vi "Process.vi"(8 "error in":errorcluster, 11 "Inst.Transport in":refnum<class "Inst.Transport.lvclass">) -> (0 "error out":errorcluster, 3 "Inst.Transport out":refnum<class "Inst.Transport.lvclass">)   [LabVIEW 2019, in "Inst.Transport.lvclass"]
doc: "---------------------------------------------------------------\nJKI State Machine Objects™\nhttp://jki.net/state-machine-objects/\nCopyright (C) 2005-2015, JKI <info@jki.net>\nALL RIGHTS RESERVED"
uses:
  Inst.Transport.lvclass
  C:/Program Files/National Instruments/LabVIEW 2019/vi.lib/JKI/JKI SMO/SMO/SMO.lvclass
  C:/Program Files/National Instruments/LabVIEW 2019/user.lib/LevyLab/Instrument Framework/Instrument/Instrument.lvclass
  Transport/Typedefs/Lockin_Sweep JSON--Cluster.ctl
  Transport/Transport.lvclass/Transport.ctl
  Typedefs/UI State--enum.ctl
  Typedefs/Inst.Transport.PublicCommands--Enum.ctl
  Typedefs/Inst.Transport.ProtectedCommands--Enum.ctl
  Typedefs/startTransport--Request--Cluster.ctl
  Transport/Typedefs/Transport.Methods--Enum.ctl
  Typedefs/PrivateEvents--MessageToProcess.ctl
  <userlib>/LevyLab/RemoteControl/RemoteControl/Typedefs/Message--Cluster.ctl
  Typedefs/Inst.Transport.Status--Enum.ctl
  Inst.Transport.lvclass/Inst.Transport.ctl
  <vilib>/JKI/JKI SMO/SMO/SMO.lvclass/SMO.ctl
  Control Experiment/Control Experiment.lvclass
  Control Experiment/Control Experiment.lvclass/Control Experiment.ctl
  Typedefs/RefreshTime--Request--Cluster.ctl
  8f0a8fc2-545a-492d-a380-fe326c3f5926.vi
  1045582e-a15c-4059-9878-8d398bb7fea9.vi
  db7760a1-0849-494e-b918-bfd2b1278472.vi
  48eb5b5f-56a5-4c0e-b192-c05c3e35427f.vi
  <vilib>/dlg_ctls.llb/Space Constant.vi
  <vilib>/AdvancedString/1D String Array to Delimited String.vi
  db7760a1-0849-494e-b918-bfd2b1278472.vi/a990f674-cb9f-4357-b763-dc53ec849aca.vi
  db7760a1-0849-494e-b918-bfd2b1278472.vi/f77cd2e4-63f0-4db9-904d-f0a5dec29833.vi
  <vilib>/JKI/JKI SMO/SMO/Private/ReftoDVR--SMO.vi
  48eb5b5f-56a5-4c0e-b192-c05c3e35427f.vi/6567f719-b543-4a92-a900-b5266b0141ae.vi
  48eb5b5f-56a5-4c0e-b192-c05c3e35427f.vi/08d46073-01b5-4855-922c-c1023ecda8fd.vi
  <vilib>/Utility/Data Type/Get Type Information.vi
  <vilib>/Utility/Data Type/Get Numeric Information.vi
  <userlib>/_OpenG.lib/lvdata/lvdata.llb/Unwrap VVariant__ogtk.vi
  <vilib>/JDP Science/JSONtext/JSON text to Variant.vi
  <userlib>/LevyLab/Instrument Framework/Instrument/API/Instrument.sendMessageToProcess (variant).vi
  <vilib>/JDP Science/JSONtext/LVClass Serializer/JSONtext LVClass Serializer.lvclass
  <userlib>/LevyLab/Instrument Framework/Instrument Types/SCPI/Instrument.SCPI.lvclass
  <userlib>/LevyLab/Instrument Framework/Instrument/Instrument.lvclass
  <userlib>/LevyLab/RemoteControl/RemoteControl/RemoteControl.lvclass
  <userlib>/LevyLab/Debug/Debug.lvlib
  <vilib>/JKI/JKI SMO/SMO/SMO.lvclass
  Transport/Transport.lvclass
  C:/Program Files/National Instruments/LabVIEW 2019/user.lib/LevyLab/Instrument Framework/Instrument Types/SCPI/Instrument.SCPI.lvclass
panel:
  in  "Tab Control":enum32{"Main", "Sweep Config", "Debug"}(tab)
  in  "startTransport":bool
  in  "stopTransport":bool
  out "Status":string
  in  "Close VI":bool
  in  "Open  VI":bool
  in  "Ring":i32(ring) items=["Continuous B Sweep"]
  in  "Experiment Folder":string="1 -  Folder Name"
  in  "Experiment Description":string="this is the experiment description"
  in  "Sweep":T1 {"sweepTables"."Table" format="%#_3p"; "sweepTables"."Ch" min=1 max=16; "sweepChannels"."Table" format="%#_1f"; "sweepChannels"."Channel" min=1 max=128; "sweepChannels"."Start" format="%#_6p"; "sweepChannels"."End" format="%#_6p"}
  out "state history":string
  out "parameters":string
  out "command":string
  out "Secret Status":string
  # "Transport Server"
  # "Inst.Transport"
  # "For instructions on how to use the JKI State Machine Objects, examples and video tutorials, visit:\nhttp://jki.net/state-machine-objects/\n\nJKI State Machine Objects™\nhttp://jki.net/state-machine-objects/\nCopyright (C) 2005-2015, JKI <info@jki.net>\nALL RIGHTS RESERVED"
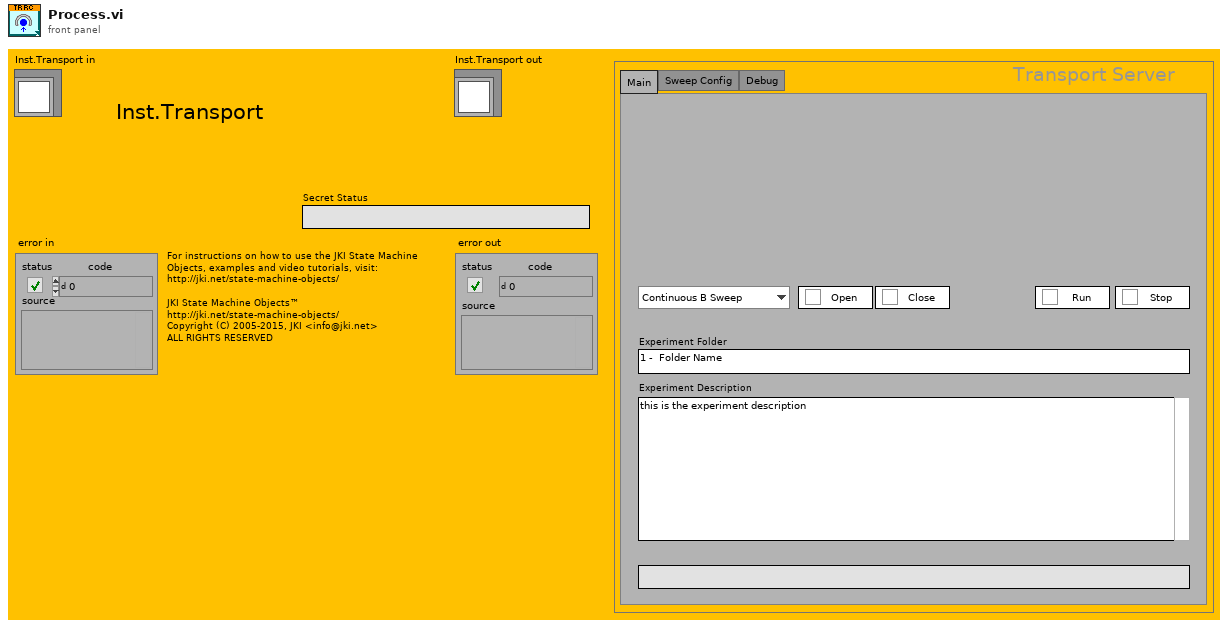
[diagram p1: front panel]
types:
  T1 = typedef "Transport.lvclass/Lockin_Sweep JSON--Cluster.ctl" = cluster{"initialWaitTime":dbl, "sweepTime":dbl, "Return to Start":bool, "sweepChannels":cluster{"Enable?":bool, "Channel":u16, "Start":dbl, "End":dbl, "Pattern":enum16{"Ramp /", "Ramp /\\", "Smooth Ramp _/", "Smooth Ramp _/\\_", "Table"}, "Table":dbl[]}[], "sweepTables":cluster{"Ch":i32, "Table":dbl[]}[]}
  T2 = typedef "Inst.Transport.lvclass/UI State--enum.ctl" = enum16{"unknown", "Opened", "Closed"}
  T3 = typedef "Inst.Transport.lvclass/Inst.Transport.ProtectedCommands--Enum.ctl" = enum16{"setStatus", "showUI", "hideUI"}
  T4 = typedef "Inst.Transport.lvclass/Inst.Transport.PublicCommands--Enum.ctl" = enum16{"startTransport", "stopTransport", "getStatus", "setExptFolder", "getExptFolder", "setExptComments", "getExptComments", "setExptParam", "appendExptParam", "clearExptParam", "setSweepConfig", "getSweepConfig", "setRefreshTime"}
  T5 = typedef "Inst.Transport.lvclass/startTransport--Request--Cluster.ctl" = cluster{"method":T6}
  T6 = typedef "Transport.lvclass/Transport.Methods--Enum.ctl" = enum16{"LockinSweep", "LockinTime", "LockinTimeDelay"}
  T7 = enum32{"invalid app kind", "Development System", "Run Time System", "Student Edition", "Embedded LabVIEW", "Evaluation", "Custom"}
  T8 = typedef "Inst.Transport.lvclass/Inst.Transport.Status--Enum.ctl" = enum16{"idle", "running"}
  T9 = enum8{"Enabled", "Disabled", "Disabled and Grayed Out"}
  T10 = enum32{"Invalid", "Standard", "Closed", "Hidden", "Minimized", "Maximized"}
  T11 = typedef "Inst.Transport.lvclass/RefreshTime--Request--Cluster.ctl" = cluster{"RefreshTime":u32}
  T12 = typedef "Inst.Transport.lvclass/PrivateEvents--MessageToProcess.ctl" = cluster{"Message":T13}
  T13 = typedef "RemoteControl.lvlib/RemoteControl.lvclass/Message--Cluster.ctl" = cluster{"Command":string, "Data":variant, "ID":string, "error":errorcluster}
  T14 = cluster{"Core":cluster{"Current VI Reference":refnum<vi>, "Close Panel on Exit?":bool, "Last Error":cluster{"error":errorcluster, "previous state":string, "remaining states":string}, "Shutdown?":bool}, "SMO":refnum<class "Inst.Transport.lvclass">, "Transport":refnum<class "Transport.lvclass">, "C.E.":refnum<class "Control Experiment.lvclass">, "Folder":string, "Comments":string, "Sweep":T1, "Status":T8, "Ring":i32, "method":T6, "methods":string[], "paths":path[], "path":path, "Running Step":i32, "sequence":string[], "MessageToProcess":T12, "UI Behavior":string, "wait":u32}
  T15 = cluster{"Current VI Reference":refnum<vi>, "Close Panel on Exit?":bool, "Last Error":cluster{"error":errorcluster, "previous state":string, "remaining states":string}, "Shutdown?":bool}
  T16 = typedef "Debug.lvlib/Attribute.Debug.lvclass/DebugBehavior.ctl" = enum16{"Normal", "Debug"}
  T17 = typedef "SMO.lvclass/Protected Events.ctl" = cluster{"StopProcesses":refnum<user-event>, "AbortProcesses":refnum<user-event>, "Config Changed":refnum<user-event>, "Dependency":refnum<user-event>}
  T18 = typedef "LV-Data.lvclass/Dictionary--cluster.ctl" = cluster{"key":string, "value":variant}
  T19 = typedef "Inst.Transport.lvclass/Inst.Transport.getAll--Cluster.ctl" = cluster{"data":variant}
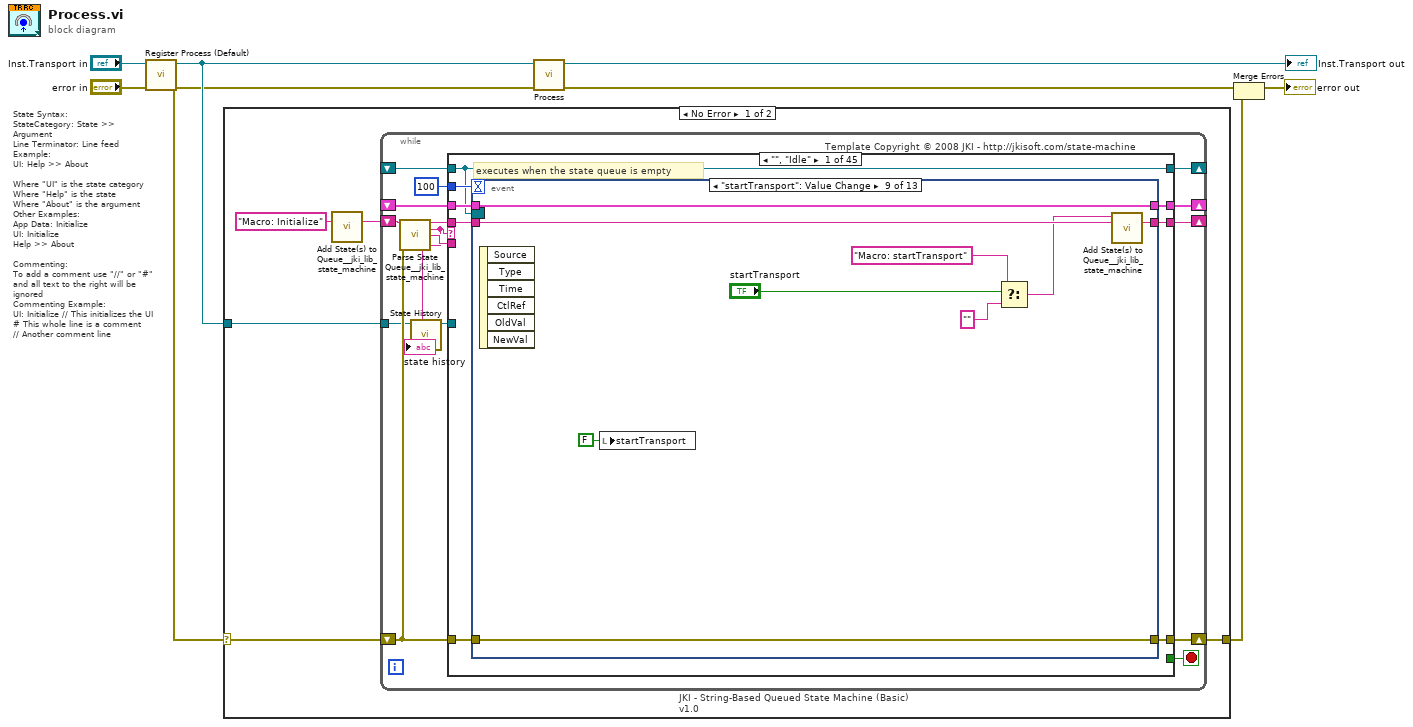
[diagram p0: block diagram]
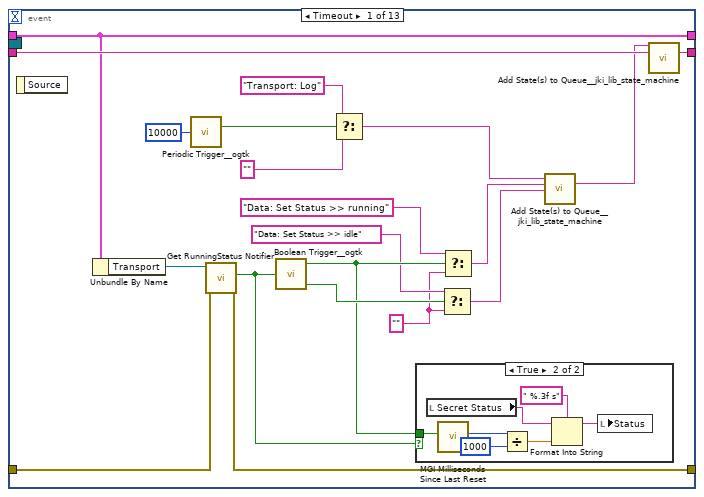
[diagram p2: hidden frame]
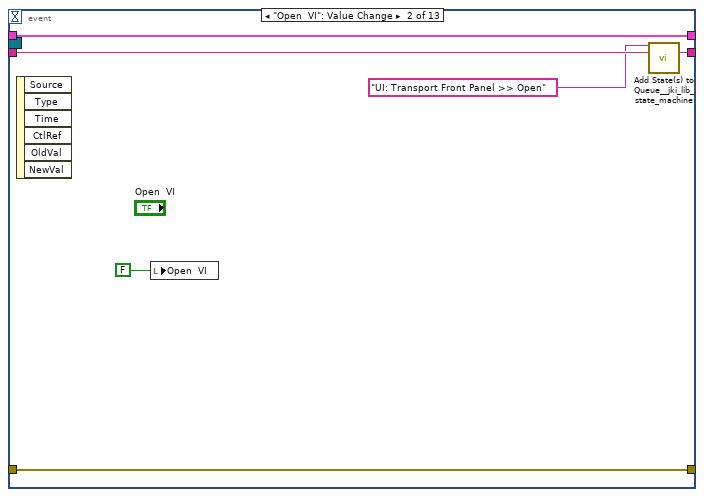
[diagram p4: hidden frame]
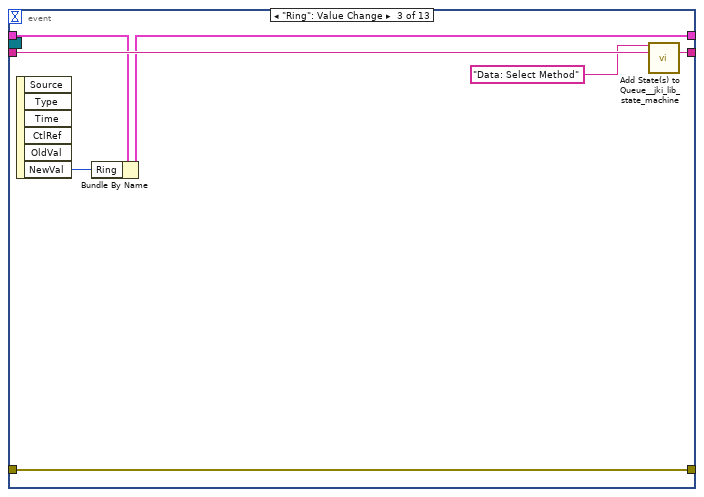
[diagram p5: hidden frame]
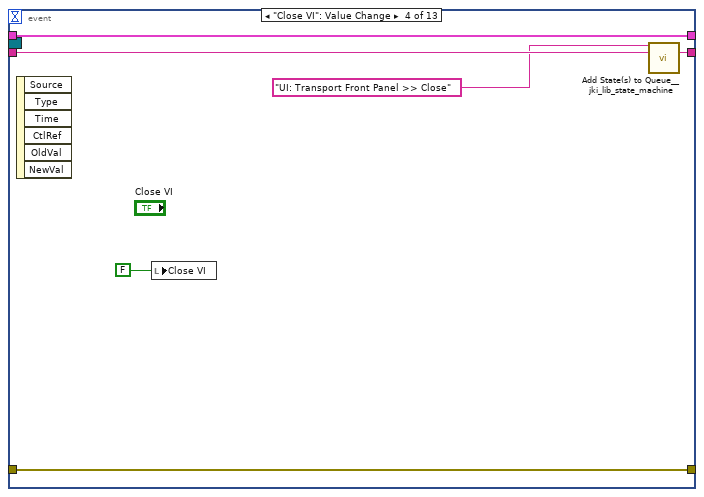
[diagram p6: hidden frame]
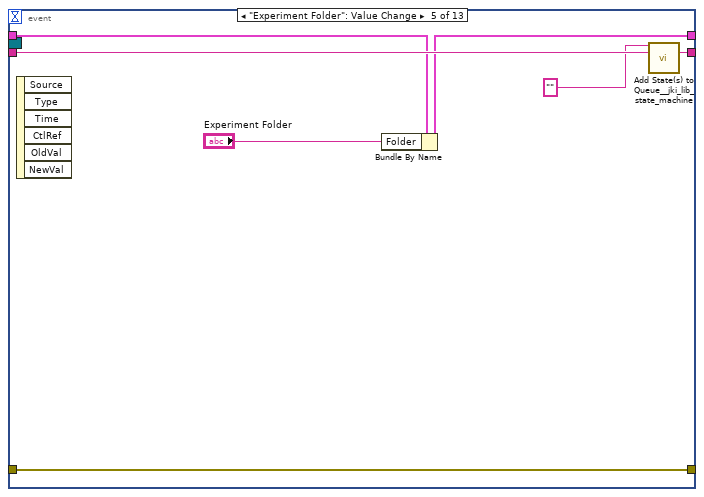
[diagram p7: hidden frame]
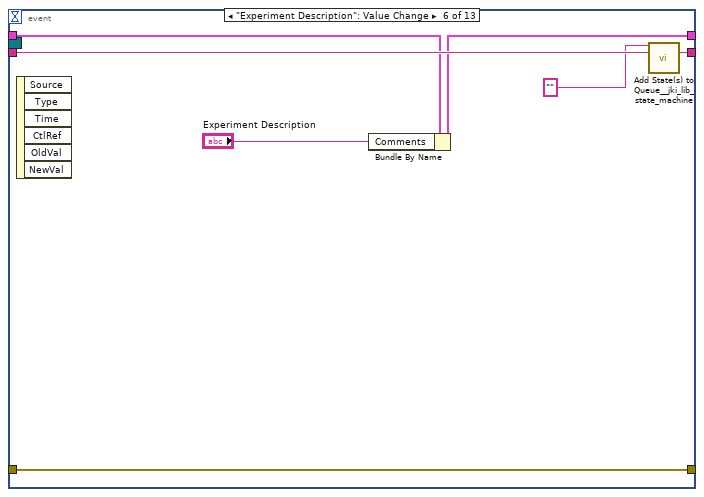
[diagram p8: hidden frame]
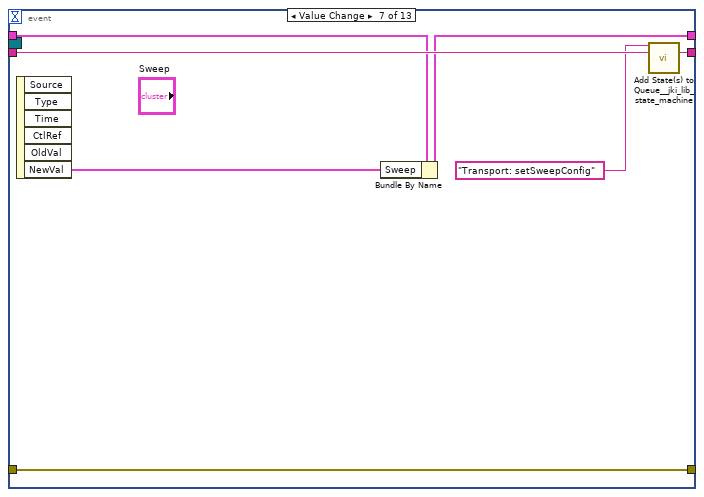
[diagram p9: hidden frame]
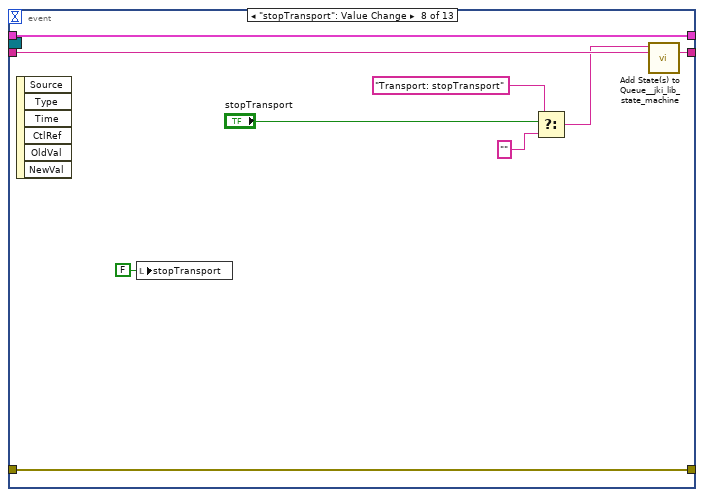
[diagram p10: hidden frame]
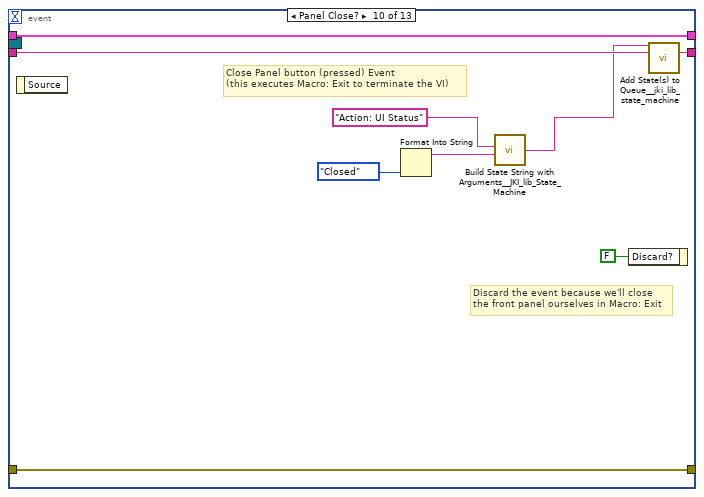
[diagram p11: hidden frame]
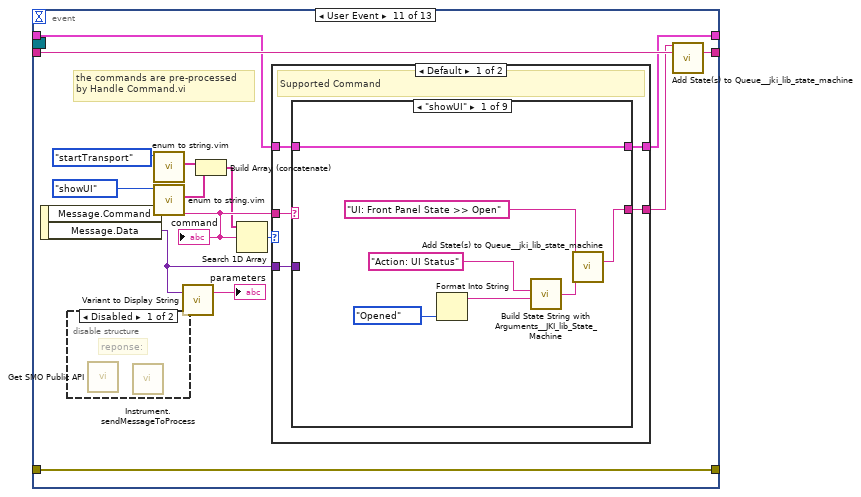
[diagram p12: hidden frame]
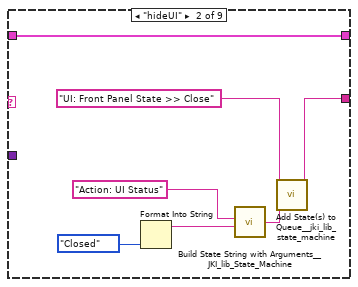
[diagram p14: hidden frame]
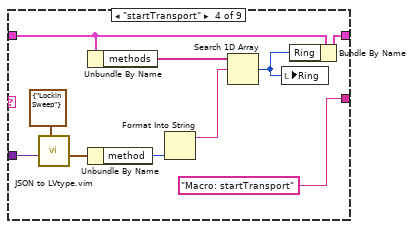
[diagram p16: hidden frame]
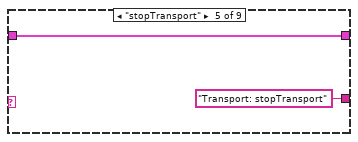
[diagram p17: hidden frame]
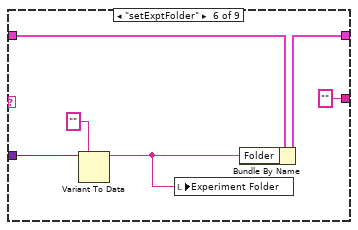
[diagram p18: hidden frame]
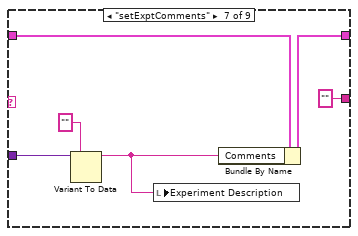
[diagram p19: hidden frame]
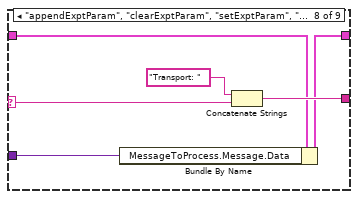
[diagram p20: hidden frame]
diagram:
  # "State Syntax:\nStateCategory: State >> Argument\nLine Terminator: Line feed\nExample:\nUI: Help >> About\n\nWhere \"UI\" is the state category\nWhere \"Help\" is the state\nWhere \"About\" is the argument\nOther Examples:\nApp Data: Initialize\nUI: Initialize\nHelp >> About\n\nCommenting:\nTo add a comment use \"//\" or \"#\" and all text to the right will be ignored\nCommenting Example:\nUI: Initialize // This initializes the UI\n# This whole line is a comment\n// Another comment line"
  n1 = call <vilib>:"Register Process (Default).vi"("error in (no error)"="error in", "SMO"="Inst.Transport in") -> ("error out"=w3:errorcluster, "SelfRef"=w6:refnum<class "Inst.Transport.lvclass">)  [unwired: 8 in]
  n2 = case shown="No Error" w3 {
    selector: w3 -> [w10 w814]
    tunnel: w6 -> [w11 _]
    tunnel: [w9 w814] -> w4
    frame No Error {
      n3 = call <vilib>:"Add State(s) to Queue__jki_lib_state_machine.vi"("State(s) in (\"\")"="Macro: Initialize") -> ("States Out"=w13:string)  [unwired: 14 in]
      n4 = while "JKI - String-Based Queued State Machine (Basic) v1.0" {
        shift-right: [w23] -> _
        shift-left: _ -> [w22]
        shift-right: [w26] -> w9
        shift-left: w10 -> [w20]
        shift-right: [w25] -> _
        shift-left: w13 -> [w27]
        tunnel: w11 -> [w14]
        shift-right: [w19] -> _
        shift-left: _ -> [w18]
        stop <- w24 stop-if-true
        # "Template Copyright © 2008 JKI - http://jkisoft.com/state-machine"
        n5 = call <vilib>:"Parse State Queue__jki_lib_state_machine.vi"("State Queue"=w27, "Error In (no error)"=w20) -> ("Remaining States"=w29:string, "Current State"=w17:string, "Arguments"=w28:string)  [unwired: 11 in]
        n6 = call <userlib>:"State History.vi"("Current State"=w17, "SMO"=w14) -> ("SMO"=w15:refnum<class "Inst.Transport.lvclass">, "History"=→"state history":string)  [unwired: 8 in]
        n7 = case shown="\"\", \"Idle\"" w17 {
          selector: w17 -> [_ _ w223 _ _ _ _ _ _ _ _ _ _ _ _ _ _ _ _ _ _ _ _ _ _ _ _ _ _ _ _ _ _ _ _ _ _ _ _ _ _ _ _ _ _]
          tunnel: w29 -> [w37 w221 w227 w246 w251 w265 w270 w294 w309 w341 w364 w380 w385 w394 w403 w410 w426 w464 w506 w515 w527 w548 w563 w574 w591 w596 w607 w614 w619 w632 w638 w646 w673 w683 w702 w715 w728 w735 w745 w759 w772 w777 w788 w794 w813]
          tunnel: w28 -> [_ _ _ _ _ _ _ _ _ w337 _ _ _ _ w395 w404 w420 w458 _ _ _ _ _ _ _ _ _ _ _ _ _ _ _ _ _ _ _ _ _ _ _ _ w781 w789 w797]
          tunnel: w22 -> [w35 w218 w225 w237 w255 w261 w267 _ w304 w326 w358 w375 w382 w392 w400 w408 w422 w457 w503 w512 w517 w538 w552 w571 w576 w593 w604 w611 w616 w625 w636 w641 w669 w680 w698 w711 w724 w730 w741 w755 w768 w774 w782 w790 w803]
          tunnel: [w34 w219 w229 w243 w256 w260 w268 w285 w306 w334 w362 w376 w383 w389 w401 w405 w423 w461 w504 w507 w525 w546 w551 w572 w579 w594 w598 w609 w617 w628 w634 w643 w648 w677 w695 w708 w721 w732 w738 w752 w766 w773 w780 w791 w805] -> w26
          tunnel: w20 -> [w33 w219 w228 w243 w257 _ w268 w285 w306 w333 w362 w377 w383 w388 w401 w406 w424 w460 w504 w507 w525 w546 w550 w572 w579 w594 w599 w608 w617 w622 w634 w643 w660 w676 w694 w705 w719 w732 w736 w754 w761 w773 w779 w791 w799]
          tunnel: [w36 w220 w226 w245 w247 w264 w269 w293 w308 w340 w363 w379 w384 w393 w402 w409 w425 w463 w505 w514 w526 w547 w562 w573 w590 w595 w606 w613 w618 w631 w637 w645 w672 w682 w701 w714 w727 w734 w744 w758 w771 w776 w787 w793 w812] -> w25
          tunnel: [_ _ _ _ _ TRUE _ _ _ _ _ _ _ _ _ _ _ _ _ _ _ _ _ _ _ _ _ _ _ _ _ _ _ _ _ _ _ _ _ _ _ _ _ _ _] -> w24
          tunnel: [w32 w218 w225 w244 w254 w261 w267 w292 w305 w327 w359 w375 w382 w392 w400 w408 w422 w457 w503 w512 w518 w539 w553 w571 w577 w593 w604 w611 w616 w625 w636 w642 w670 w680 w699 w712 w725 w731 w742 w756 w769 w774 w782 w790 w802] -> w23
          tunnel: 100 ("Timeout") -> [w31 _ _ _ _ _ _ _ _ _ _ _ _ _ _ _ _ _ _ _ _ _ _ _ _ _ _ _ _ _ _ _ _ _ _ _ _ _ _ _ _ _ _ _ _]
          tunnel: w15 -> [_ _ _ _ _ _ _ w286 _ _ _ _ _ _ _ _ _ _ _ _ _ _ _ _ _ _ _ _ _ _ _ _ _ _ _ _ _ _ _ _ _ _ _ _ _]
          tunnel: [w30 w217 w222 w234 w259 w262 w266 w291 w307 w339 w361 w374 w381 w391 w399 w407 w419 w462 w502 w513 w524 w545 w561 w570 w585 w592 w605 w612 w615 w630 w635 w644 w671 w681 w700 w713 w726 w733 w743 w757 w770 w775 w786 w792 w811] -> w19
          tunnel: w18 -> [w30 w217 w222 w234 w259 w262 w266 w291 w307 w339 w361 w374 w381 w391 w399 w407 w419 w462 w502 w513 w524 w545 w561 w570 w585 w592 w605 w612 w615 _ w635 w644 w671 w681 w700 w713 w726 w733 w743 w757 w770 w775 w786 w792 w811]
          frame "", "Idle" {
            # "executes when the state queue is empty"
            n8 = event shown="[8] \"startTransport\": Value Change" {
              selector: w30 -> [_ _ _ _ _ _ _ _ _ _ _ _ _]
              dyn-events: _ -> [_ _ _ _ _ _ _ _ _ _ _ _ _]
              timeout: w31 -> [_ _ _ _ _ _ _ _ _ _ _ _ _]
              tunnel: w37 -> [w57 w70 w77 w83 w90 w97 w104 w113 w122 w131 w146 w211 w216]
              tunnel: [w56 w69 w76 w82 w89 w96 w103 w112 w121 w130 w145 w210 w215] -> w36
              tunnel: w35 -> [w51 w67 w73 w80 w84 w92 w99 w110 w119 w128 w140 w208 w213]
              tunnel: [w49 w68 w75 w81 w88 w95 w102 w105 w115 w129 w144 w209 w214] -> w34
              tunnel: w33 -> [w48 w68 w75 w81 w88 w95 w102 w105 w115 w129 w144 w209 w214]
              tunnel: [w51 w67 w72 w80 w85 w93 w100 w110 w119 w128 w139 w208 w213] -> w32
              event Timeout {
                w38 = ""
                n9 = event-data() -> ()  [unwired: 1 in, 1 out]
                n10 = Unbundle By Name(w51) -> ("Transport"=w50:refnum<class "Transport.lvclass">)
                n11 = call <userlib>:"Periodic Trigger__ogtk.vi"("time (ms)"=u32 10000) -> ("Triggered"=w54:bool)  [unwired: 12 in, 2 out]
                n12 = call "Get RunningStatus Notifier.vi"("error in (no error)"=w48, "Transport in"=w50) -> ("error out"=w49:errorcluster, "Running?"=w41:bool)  [unwired: 7 in, 1 out]
                n13 = call <userlib>:"Boolean Trigger__ogtk.vi"("Boolean Input"=w41) -> ("Rising Edge"=w42:bool, "Falling Edge"=w47:bool)  [unwired: 1 in]
                n14 = Select(t="Transport: Log", s=w54, f="") -> (s? t:f=w45:string)
                n15 = case shown="True" w41 {
                  tunnel: w42 -> [_ w64]
                  frame False {
                  }
                  frame True {
                    n16 = local read "Secret Status"() -> (w61:string)
                    n17 = call <userlib>:"MGI Milliseconds Since Last Reset.vi"("Reset (F)"=w64) -> ("ms"=w60:u32)  [unwired: 5 in, 1 out]
                    n18 = Divide(x=w60, y=u32 1000) -> (x/y=w58:dbl)
                    n19 = Format Into String(format string=" %.3f s", initial string=w61, w58) -> (resulting string=w63:string)  [unwired: 1 in, 1 out]
                    n20 = local write "Status"(w63) -> ()
                  }
                }
                n21 = Select(t="Data: Set Status >> idle", s=w47, f=w38) -> (s? t:f=w40:string)
                n22 = Select(t="Data: Set Status >> running", s=w42, f=w38) -> (s? t:f=w44:string)
                n23 = call <vilib>:"Add State(s) to Queue__jki_lib_state_machine.vi"("State(s) in Front (\"\")"=w45, "State(s) in (\"\")"=w44, "State(s) at Back (\"\")"=w40) -> ("States Out"=w43:string)  [unwired: 12 in]
                n24 = call <vilib>:"Add State(s) to Queue__jki_lib_state_machine.vi"("State(s) in Front (\"\")"=w43, "State(s) in (\"\")"=w57) -> ("States Out"=w56:string)  [unwired: 13 in]
              }
              event "Open  VI": Value Change {
                n25 = event-data() -> ()  [unwired: 1 in, 6 out]
                n26 = local write "Open  VI"(FALSE ("Open VI")) -> ()
                n27 = call <vilib>:"Add State(s) to Queue__jki_lib_state_machine.vi"("State(s) in Front (\"\")"="UI: Transport Front Panel >> Open" ("State(s) in Front (\"\")"), "State(s) in (\"\")"=w70) -> ("States Out"=w69:string)  [unwired: 13 in]
              }
              event "Ring": Value Change {
                n28 = event-data() -> ("NewVal"=w71:i32)  [unwired: 1 in, 5 out]
                n29 = Bundle By Name(cluster=w73, "Ring"=w71) -> (w72:T14)
                n30 = call <vilib>:"Add State(s) to Queue__jki_lib_state_machine.vi"("State(s) in Front (\"\")"="Data: Select Method" ("State(s) in Front (\"\")"), "State(s) in (\"\")"=w77) -> ("States Out"=w76:string)  [unwired: 13 in]
              }
              event "Close VI": Value Change {
                n31 = event-data() -> ()  [unwired: 1 in, 6 out]
                n32 = local write "Close VI"(FALSE ("Open VI")) -> ()
                n33 = call <vilib>:"Add State(s) to Queue__jki_lib_state_machine.vi"("State(s) in Front (\"\")"="UI: Transport Front Panel >> Close" ("State(s) in Front (\"\")"), "State(s) in (\"\")"=w83) -> ("States Out"=w82:string)  [unwired: 13 in]
              }
              event "Experiment Folder": Value Change {
                n34 = event-data() -> ()  [unwired: 1 in, 6 out]
                n35 = Bundle By Name(cluster=w84, "Folder"="Experiment Folder") -> (w85:T14)
                n36 = call <vilib>:"Add State(s) to Queue__jki_lib_state_machine.vi"("State(s) in Front (\"\")"="" ("State(s) in Front (\"\")"), "State(s) in (\"\")"=w90) -> ("States Out"=w89:string)  [unwired: 13 in]
              }
              event "Experiment Description": Value Change {
                n37 = event-data() -> ()  [unwired: 1 in, 6 out]
                n38 = Bundle By Name(cluster=w92, "Comments"="Experiment Description") -> (w93:T14)
                n39 = call <vilib>:"Add State(s) to Queue__jki_lib_state_machine.vi"("State(s) in Front (\"\")"="" ("State(s) in Front (\"\")"), "State(s) in (\"\")"=w97) -> ("States Out"=w96:string)  [unwired: 13 in]
              }
              event Value Change {
                n40 = event-data() -> ("NewVal"=w98:T1)  [unwired: 1 in, 5 out]
                n41 = Bundle By Name(cluster=w99, "Sweep"=w98) -> (w100:T14)
                n42 = call <vilib>:"Add State(s) to Queue__jki_lib_state_machine.vi"("State(s) in Front (\"\")"="Transport: setSweepConfig" ("State(s) in Front (\"\")"), "State(s) in (\"\")"=w104) -> ("States Out"=w103:string)  [unwired: 13 in]
              }
              event "stopTransport": Value Change {
                n43 = event-data() -> ()  [unwired: 1 in, 6 out]
                n44 = local write "stopTransport"(FALSE ("Open VI")) -> ()
                n45 = Select(t="Transport: stopTransport" ("State(s) in Front (\"\")"), s="stopTransport", f="") -> (s? t:f=w107:string)
                n46 = call <vilib>:"Add State(s) to Queue__jki_lib_state_machine.vi"("State(s) in Front (\"\")"=w107, "State(s) in (\"\")"=w113) -> ("States Out"=w112:string)  [unwired: 13 in]
              }
              event "startTransport": Value Change {
                n47 = event-data() -> ()  [unwired: 1 in, 6 out]
                n48 = local write "startTransport"(FALSE ("Open VI")) -> ()
                n49 = Select(t="Macro: startTransport" ("State(s) in Front (\"\")"), s="startTransport", f="") -> (s? t:f=w116:string)
                n50 = call <vilib>:"Add State(s) to Queue__jki_lib_state_machine.vi"("State(s) in Front (\"\")"=w116, "State(s) in (\"\")"=w122) -> ("States Out"=w121:string)  [unwired: 13 in]
              }
              event Panel Close? {
                # "Discard the event because we'll close the front panel ourselves in Macro: Exit"
                # "Close Panel button (pressed) Event\n(this executes Macro: Exit to terminate the VI)"
                n51 = event-data() -> ()  [unwired: 1 in, 1 out]
                n52 = Format Into String(UI_State--enum."Closed" ("UI State")) -> (resulting string=w123:string)  [unwired: 3 in, 1 out]
                n53 = call <vilib>:"Build State String with Arguments__JKI_lib_State_Machine.vi"("Arguments (\"\")"=w123, "State"="Action: UI Status" ("f")) -> ("State with Arguments"=w125:string)  [unwired: 4 in]
                n54 = event-data("Discard?"=FALSE) -> ()  [unwired: 1 in, 1 out]
                n55 = call <vilib>:"Add State(s) to Queue__jki_lib_state_machine.vi"("State(s) in Front (\"\")"=w125, "State(s) in (\"\")"=w131) -> ("States Out"=w130:string)  [unwired: 13 in]
              }
              event User Event {
                # "the commands are pre-processed\nby Handle Command.vi"
                n56 = event-data() -> ("Message.Command"=w138:string, "Message.Data"=w136:variant)  [unwired: 1 in]
                "command" <- w138
                n57 = disable-structure shown="Disabled" {
                  frame Disabled {
                    # "reponse:"
                    n58 = call-dynamic "Get SMO Public API.vi"() -> ()  [unwired: 9 in, 3 out]
                    n59 = call-poly <userlib>:"Instrument.sendMessageToProcess.vi"() -> ()  [unwired: 10 in, 2 out]
                  }
                  frame Enabled {
                  }
                }
                n60 = call "enum to string.vim"("enum in"=Inst.Transport.PublicCommands--Enum."startTransport" ("PublicCommands")) -> ("strings out"=w133:string[])  [unwired: 9 in, 1 out]
                n61 = call "enum to string.vim"("enum in"=Inst.Transport.ProtectedCommands--Enum."showUI" ("ProtectedCommands")) -> ("strings out"=w134:string[])  [unwired: 9 in, 1 out]
                n62 = call "Variant to Display String.vi"("Variant"=w136) -> ("xml string"=→"parameters":string)  [unwired: 2 in]
                n63 = Build Array (concatenate)(w133, w134) -> (w132:string[])
                n64 = Search 1D Array(1D array=w132, element=w138) -> (index of element=w143:i32)  [unwired: 1 in]
                n65 = case shown="Default" w143 {
                  tunnel: [w151 "" ("Empty String Constant")] -> w142
                  tunnel: w138 -> [w150 _]
                  tunnel: w136 -> [w149 _]
                  tunnel: w140 -> [w148 w205]
                  tunnel: [w147 w205] -> w139
                  frame Default {
                    # "Supported Command"
                    n66 = case shown="\"showUI\"" w150 {
                      selector: w150 -> [_ _ _ _ _ _ _ w195 w204]
                      tunnel: [w152 w159 _ "Macro: startTransport" "Transport: stopTransport" ("State with Arguments") "" ("State with Arguments") "" ("State with Arguments") w194 w203] -> w151
                      tunnel: w149 -> [_ _ _ w174 _ w180 w187 w191 w199]
                      tunnel: w148 -> [w158 w165 w166 w172 w178 w184 w190 w192 w201]
                      tunnel: [w158 w165 w166 w176 w178 w183 w189 w193 w202] -> w147
                      frame "showUI" {
                        n67 = Format Into String(UI_State--enum."Opened" ("UI State")) -> (resulting string=w155:string)  [unwired: 3 in, 1 out]
                        n68 = call <vilib>:"Build State String with Arguments__JKI_lib_State_Machine.vi"("Arguments (\"\")"=w155, "State"="Action: UI Status" ("f")) -> ("State with Arguments"=w154:string)  [unwired: 4 in]
                        n69 = call <vilib>:"Add State(s) to Queue__jki_lib_state_machine.vi"("State(s) in Front (\"\")"="UI: Front Panel State >> Open" ("State with Arguments"), "State(s) at Back (\"\")"=w154) -> ("States Out"=w152:string)  [unwired: 13 in]
                      }
                      frame "hideUI" {
                        n70 = Format Into String(UI_State--enum."Closed" ("UI State")) -> (resulting string=w162:string)  [unwired: 3 in, 1 out]
                        n71 = call <vilib>:"Build State String with Arguments__JKI_lib_State_Machine.vi"("Arguments (\"\")"=w162, "State"="Action: UI Status" ("f")) -> ("State with Arguments"=w161:string)  [unwired: 4 in]
                        n72 = call <vilib>:"Add State(s) to Queue__jki_lib_state_machine.vi"("State(s) in Front (\"\")"="UI: Front Panel State >> Close" ("State with Arguments"), "State(s) at Back (\"\")"=w161) -> ("States Out"=w159:string)  [unwired: 13 in]
                      }
                      frame Default {
                      }
                      frame "startTransport" {
                        n73 = call "JSON to LVtype.vim"("type"=T5 {"method"=enum."LockinSweep"} ("startTransport"), "JSON Data in"=w174) -> ("Data out"=w173:T5)  [unwired: 8 in, 1 out]
                        n74 = Unbundle By Name(w172) -> ("methods"=w170:string[])
                        n75 = Unbundle By Name(w173) -> ("method"=w169:T6)
                        n76 = Format Into String(w169) -> (resulting string=w171:string)  [unwired: 3 in, 1 out]
                        n77 = Search 1D Array(1D array=w170, element=w171) -> (index of element=w168:i32)  [unwired: 1 in]
                        n78 = local write "Ring"(w168) -> ()
                        n79 = Bundle By Name(cluster=w172, "Ring"=w168) -> (w176:T14)
                      }
                      frame "stopTransport" {
                      }
                      frame "setExptFolder" {
                        n80 = Variant To Data(type="", Variant=w180) -> (data=w179:string)  [unwired: 1 in, 1 out]
                        n81 = local write "Experiment Folder"(w179) -> ()
                        n82 = Bundle By Name(cluster=w184, "Folder"=w179) -> (w183:T14)
                      }
                      frame "setExptComments" {
                        n83 = Variant To Data(type="", Variant=w187) -> (data=w185:string)  [unwired: 1 in, 1 out]
                        n84 = local write "Experiment Description"(w185) -> ()
                        n85 = Bundle By Name(cluster=w190, "Comments"=w185) -> (w189:T14)
                      }
                      frame "appendExptParam", "clearExptParam", "setExptParam", "setRefreshTime" {
                        n86 = Bundle By Name(cluster=w192, "MessageToProcess.Message.Data"=w191) -> (w193:T14)
                        n87 = Concatenate Strings("Transport: ", w195) -> (w194:string)
                      }
                      frame "setSweepConfig" {
                        n88 = Variant To Data(type=T1 {"initialWaitTime"=0.0, "sweepTime"=0.0, "Return to Start"=FALSE, "sweepChannels"=[], "sweepTables"=[]} ("Lockin_Sweep"), Variant=w199) -> (data=w197:T1)  [unwired: 1 in, 1 out]
                        n89 = Bundle By Name(cluster=w201, "Sweep"=w197) -> (w202:T14)
                        n90 = local write "Sweep"(w197) -> ()
                        n91 = Concatenate Strings("Transport: ", w204) -> (w203:string)
                      }
                    }
                  }
                  frame -1 {
                    # "Return Error?"
                    # "Command Not Found"
                  }
                }
                n92 = call <vilib>:"Add State(s) to Queue__jki_lib_state_machine.vi"("State(s) in Front (\"\")"=w142, "State(s) in (\"\")"=w146) -> ("States Out"=w145:string)  [unwired: 13 in]
              }
              event User Event {
                n93 = event-data() -> ()  [unwired: 1 in, 5 out]
                n94 = call <vilib>:"Add State(s) to Queue__jki_lib_state_machine.vi"("State(s) in Front (\"\")"="Macro: Exit", "State(s) in (\"\")"=w211) -> ("States Out"=w210:string)  [unwired: 13 in]
              }
              event User Event {
                # "On Abort, no nice macro exit, but exit right away"
                n95 = event-data() -> ()  [unwired: 1 in, 5 out]
                n96 = call <vilib>:"Add State(s) to Queue__jki_lib_state_machine.vi"("State(s) in Front (\"\")"="Exit", "State(s) in (\"\")"=w216) -> ("States Out"=w215:string)  [unwired: 13 in]
              }
            }
          }
          frame "---------- Core ----------" {
            # "Do not put any code in this frame.\n(it is a separator no-op)"
            n97 = call <vilib>:"Add State(s) to Queue__jki_lib_state_machine.vi"("State(s) in (\"\")"=w221) -> ("States Out"=w220:string)  [unwired: 14 in]
          }
          frame Default {
            w232 = 42 items=["No error", "Argument error", "Memory is full", "Out of zone", "End of file", "File already open", "Generic file I/O error", "File not found", "File permission error", "Disk is full", "Duplicate path", "Too many files open", "System feature not enabled", "Resource file not found", "Cannot add resource", "Resource not found", "Image not found", "Image memory error", "Pen does not exist", "Config type invalid", "Config token not found", "Config parse error", "Config memory error", "Bad external code format", "Bad external code offset", "External code not present", "Null window", "Destroy window error", "Null menu", "Print aborted", "Bad print record", "Print driver error", "Windows error during printing", "Memory error during printing", "Print dialog error", "Generic print error", "Invalid device refnum", "Device not found", "Device parameter error", "Device unit error", "Cannot open device", "Device call aborted", "Generic error", "Cancelled by user", "Object ID too low", "Object ID too high", "Object not in heap", "Unknown heap", "Unknown object (invalid DefProc)", "Unknown object (DefProc not in table)", "Message out of range", "Invalid (null) method", "Unknown message", "Manager call not supported", "Bad address", "Network operation in progress", "Network operation timed out", "Connection is busy", "Network attribute not supported", "Network error", "Address in use", "System out of memory", "Connection aborted", "Connection refused", "Not connected", "Already connected", "Connection closed", "Initialization error (interapplication manager)", "Bad occurrence", "Wait on unbound occurrence handler", "Occurrence queue overflow", "Datalog type conflict", "Unused", "Unrecognized type (interapplication manager)", "Memory corrupt", "Failed to make temporary DLL", "Old CIN version", "Drag socket not found", "Failed to load drop-object", "Failed to register OLE object", "Failed to release OLE object", "Format specifier type mismatch", "Unknown format specifier", "Too few format specifiers", "Too many format specifiers", "Scan failed", "Newer CIN version", "Error converting to variant", "Runtime menu error", "Password tampered", "Variant attribute not found", "Incompatible variant data type", "Event data is not available", "Event Store is not present", "Occurrence is not found", "Event Queue is not created", "Event info is not available", "Refnum passed is NULL", "Error retrieving Class GUID", "Error retrieving CoClass GUID", "Error retrieving TypeLib GUID.", "Bad built application magic bytes.", "Specific driver is different from the specific driver associated with the Logical Name.", "There is no session opened to the class driver.", "Max Error", "MAX - Error with config objects", "MAX - Error loading configuration", "MAX - Group not supported"]
            # "Current State"
            # "Do not delete, rename, or modify this frame.\n(this is used to capture unhandled states and typos)"
            # "Handle mistyped state name (developer tool)"
            n98 = Format Into String(format string="Software Exception: Unhandled State \"%s\"." ("message"), error in=w228, w223) -> (resulting string=w231:string, error out=w230:errorcluster)  [unwired: 1 in]
            n99 = call <vilib>:"Error Cluster From Error Code.vi"("show call chain? (False)"=TRUE, "error in (no error)"=w230, "error message (\"\")"=w231, "error code (0)"=w232) -> ("error out"=w229:errorcluster)  [unwired: 5 in]
            n100 = call <vilib>:"Add State(s) to Queue__jki_lib_state_machine.vi"("State(s) in (\"\")"=w227) -> ("States Out"=w226:string)  [unwired: 14 in]
          }
          frame "Initialize Core Data" {
            # "Do not delete, rename, or modify this frame.\n(this is used to determine panel behavior on exit)"
            # "originally closed?"
            # "exe?"
            # "If panel starts closed or is an EXE, then close it when we exit"
            n101 = property class="VI"() -> ("Front Panel.Open"=w242:bool)  [unwired: 2 in, 2 out]
            n102 = property class="App"() -> ("App.Kind"=w241:T7)  [unwired: 2 in, 2 out]
            n103 = control-ref of="Current VI Reference"() -> (w235:refnum<vi>)
            n104 = Not(x=w242) -> (.not. x?=w239:bool)
            n105 = Equal?(x=w241, y=T7."Run Time System" ("Application:Kind")) -> (x = y?=w238:bool)
            n106 = Or(x=w239, y=w238) -> (x .or. y?=w236:bool)
            n107 = Bundle By Name(cluster=w237, "Core.Current VI Reference"=w235, "Core.Close Panel on Exit?"=w236) -> (w244:T14)
            n108 = call <vilib>:"Add State(s) to Queue__jki_lib_state_machine.vi"("State(s) in (\"\")"=w246) -> ("States Out"=w245:string)  [unwired: 14 in]
          }
          frame "Error Handler" {
            w252 = FALSE  # Stop on Unhandled Error (T)
            w256 = errorcluster {"status"=FALSE, "code"=0, "source"=""}  # error out
            # "clear error"
            # "There was an error while handling the error.\nStop the process. This error can only occur if public events references are invalid or if the state machine object is destroyed."
            # "Overwrite this method to handle errors and pass to parent if not handled. Parent will fire a public event if the error is not handled up the chain of classes."
            n109 = Unbundle By Name(w255) -> ("SMO"=w258:refnum<class "Inst.Transport.lvclass">)
            n110 = call-dynamic "Handle Error.vi"("Stop on Unhandled Error (T)"=w252, "error in"=w257, "SMO"=w258) -> ("handling error"=w248:errorcluster, "Unhandled error"=w253:errorcluster)  [unwired: 6 in, 1 out]
            n111 = Bundle By Name(cluster=w255, "Core.Last Error.remaining states"=w251, "Core.Last Error.error"=w253) -> (w254:T14)
            n112 = Select(t="Exit", s=w248, f="Macro: Post Error Handling") -> (s? t:f=w247:string)
          }
          frame "Exit" {
            # "Do not put any code in this frame.\n(No errors that occur here will be handled.)"
            n113 = Unbundle By Name(w261) -> ("Core.Last Error.error"=w260:errorcluster)
            n114 = call <vilib>:"Add State(s) to Queue__jki_lib_state_machine.vi"("State(s) in (\"\")"=w265) -> ("States Out"=w264:string)  [unwired: 14 in]
          }
          frame "---------- Data ----------" {
            # "Do not put any code in this frame.\n(It is a separator no-op. You can make a copy of this frame to create a new Data frame)"
            n115 = call <vilib>:"Add State(s) to Queue__jki_lib_state_machine.vi"("State(s) in (\"\")"=w270) -> ("States Out"=w269:string)  [unwired: 14 in]
          }
          frame "Data: Initialize" {
            w273 = string[] []  # methods
            w274 = 0  # Ring
            w275 = Inst.Transport.Status--Enum."idle"  # Status
            w276 = path ""  # path
            w277 = path[] []  # paths
            w271 = Transport.Methods--Enum."LockinSweep"  # method
            w283 = u32 0  # wait
            w284 = ""  # UI Behavior
            w287 = T12 {"Message"={"Command"="", "Data"=variant(string ""), "ID"="", "error"={"status"=FALSE, "code"=0, "source"=""}}}  # MessageToProcess
            w288 = string[] []  # sequence
            w289 = -1  # Running Step
            w290 = T15 {"Current VI Reference"=refnum, "Close Panel on Exit?"=FALSE, "Last Error"={"error"={"status"=FALSE, "code"=0, "source"=""}, "previous state"="", "remaining states"=""}, "Shutdown?"=FALSE}  # Core
            # "do not delete - used by framework"
            # "Initialize the shift-register data, here.\n(data names are defined by what you wire into the bundle function)"
            n116 = Unbundle By Name(w286) -> ("Transport"=w278:refnum<class "Transport.lvclass">, "Folder"=w280:string, "Comments"=w279:string, "Sweep"=w272:T1)
            n117 = call "Read Dependencies.vi"("Transport"=w278) -> ("C.E."=w281:refnum<class "Control Experiment.lvclass">, "Transport"=w282:refnum<class "Transport.lvclass">)  [unwired: 8 in, 1 out]
            n118 = Bundle("Core"=w290, "SMO"=w286, "Transport"=w282, "C.E."=w281, "Folder"=w280, "Comments"=w279, "Sweep"=w272, "Status"=w275, "Ring"=w274, "method"=w271, "methods"=w273, "paths"=w277, "path"=w276, "Running Step"=w289, "sequence"=w288, "MessageToProcess"=w287, "UI Behavior"=w284, "wait"=w283) -> (w292:T14)  [unwired: 1 in]
            n119 = call <vilib>:"Add State(s) to Queue__jki_lib_state_machine.vi"("State(s) in (\"\")"=w294) -> ("States Out"=w293:string)  [unwired: 14 in]
          }
          frame "Data: Populate Ring" {
            n120 = call "Application user.lib.vi"() -> ("path out"=w297:path)  [unwired: 10 in, 1 out]
            n121 = call <vilib>:"Delimited String to 1D String Array.vi"("delimiter"="\n" ("delimiter (Tab)"), "delimited string"="Lockin_sweep.vi\nLockin_time.vi\nTHz_TimeDelay.vi\nSweep Control.vi\nContinuous B Sweep.vi") -> ("string array"=w301:string[])  [unwired: 9 in]
            n122 = call <vilib>:"Delimited String to 1D String Array.vi"("delimiter"="\n" ("delimiter (Tab)"), "delimited string"="LockinSweep\nLockinTime\nLockinTimeDelay\nSweep Control\nContinuous B Sweep") -> ("string array"=w299:string[])  [unwired: 9 in]
            n123 = for {
              tunnel: [w312] -> w302 mode=indexing if=w313
              tunnel: [w317] -> w295 mode=indexing if=w313
              tunnel: w299 -> [w317] mode=indexing
              tunnel: w301 -> [w316] mode=indexing
              tunnel: w297 -> [w315]
              n124 = call <vilib>:"Recursive File List.vi"("pattern"=w316, "Folder Path"=w315) -> ("All Files in Dir"=w314:path[])  [unwired: 5 in, 4 out]
              n125 = Index Array(array=w314) -> (element=w311:path)  [unwired: 1 in]
              n126 = Empty String/Path?(string/path=w311) -> (empty?=w310:bool)
              n127 = case shown="False" w310 {
                tunnel: [w320 FALSE ("file or folder exists?")] -> w313
                tunnel: [w319 w322] -> w312
                tunnel: w311 -> [w318 w322]
                frame False {
                  n128 = call <vilib>:"Check if File or Folder Exists.vi"("path"=w318) -> ("file or folder exists?"=w320:bool, "dup path"=w319:path)  [unwired: 8 in, 1 out]
                }
                frame True {
                }
              }
            }
            n129 = Bundle By Name(cluster=w304, "paths"=w302, "methods"=w295) -> (w305:T14)
            n130 = property on="Ring" class="Ring (strict)"("Strings []"=w295) -> ()  [unwired: 2 in, 2 out]
            n131 = call <vilib>:"Add State(s) to Queue__jki_lib_state_machine.vi"("State(s) in (\"\")"=w309) -> ("States Out"=w308:string)  [unwired: 14 in]
          }
          frame "Data: Set Status" {
            # "Dat: Set Status.\n()"
            n132 = Unbundle By Name(w326) -> ("SMO"=w335:refnum<class "Inst.Transport.lvclass">, "methods"=w324:string[], "Ring"=w325:i32)
            n133 = Scan From String(input string=w337, default 1=Inst.Transport.Status--Enum."running" ("Status")) -> (output 1=w328:T8)  [unwired: 3 in, 3 out]
            n134 = Index Array(array=w324, index=w325) -> (element=w323:string)
            n135 = case shown="\"running\"" w328 {
              selector: w328 -> [_ w345]
              tunnel: ["" w348] -> w330
              tunnel: w323 -> [_ w346]
              tunnel: [TRUE ("Visible") TRUE ("Visible")] -> w329
              frame "idle", Default {
              }
              frame "running" {
                n136 = Format Into String(format string="%s: %s", w346, w345) -> (resulting string=w348:string)  [unwired: 2 in, 1 out]
              }
            }
            n137 = property on="stopTransport" class="Bool (strict)"("Visible"=w329) -> ()  [unwired: 2 in, 2 out]
            n138 = call <vilib>:"Build State String with Arguments__JKI_lib_State_Machine.vi"("Arguments (\"\")"=w330, "State"="Action: Status") -> ("State with Arguments"=w332:string)  [unwired: 4 in]
            n139 = call-poly <userlib>:"Instrument.sendMessageToProcess.vi"("error in (no error)"=w333, "Data"=w328, "Command"=Inst.Transport.ProtectedCommands--Enum."setStatus" ("ProtectedCommands"), "Instrument"=w335) -> ("error out"=w334:errorcluster)  [unwired: 6 in, 1 out]
            n140 = Bundle By Name(cluster=w326, "Status"=w328) -> (w327:T14)
            n141 = call <vilib>:"Add State(s) to Queue__jki_lib_state_machine.vi"("State(s) in Front (\"\")"=w332, "State(s) in (\"\")"=w341) -> ("States Out"=w340:string)  [unwired: 13 in]
          }
          frame "Data: Select Method" {
            # "Do not put any code in this frame.\n(It is a separator no-op. You can make a copy of this frame to create a new Data frame)"
            n142 = Unbundle By Name(w358) -> ("methods"=w360:string[], "Ring"=w357:i32, "method"=w356:T6)
            n143 = Index Array(array=w360, index=w357) -> (element=w351:string)
            n144 = call <vilib>:"Delimited String to 1D String Array.vi"("delimiter"="\n" ("delimiter (Tab)"), "delimited string"="LockinSweep\nLockinTime\nLockinTimeDelay") -> ("string array"=w352:string[])  [unwired: 9 in]
            n145 = Search 1D Array(1D array=w352, element=w351) -> (index of element=w353:i32)  [unwired: 1 in]
            n146 = Greater Or Equal To 0?(x=w353) -> (x >= 0?=w350:bool)
            n147 = case shown="True" w350 {
              tunnel: [w365 w373] -> w359
              tunnel: w358 -> [w365 w372]
              tunnel: w356 -> [_ w371]
              tunnel: w351 -> [_ w368]
              tunnel: [T9."Disabled and Grayed Out" ("Disabled") T9."Enabled" ("Disabled")] -> w349
              frame False {
              }
              frame True {
                n148 = Scan From String(input string=w368, default 1=w371) -> (error out=w369:errorcluster, output 1=w370:T6)  [unwired: 3 in, 2 out]
                n149 = call <vilib>:"Clear Errors.vi"("error in (no error)"=w369) -> ()  [unwired: 5 in, 2 out]
                n150 = Bundle By Name(cluster=w372, "method"=w370) -> (w373:T14)
              }
            }
            n151 = property on="startTransport" class="Bool (strict)"("DisabledEnum"=w349) -> ()  [unwired: 2 in, 2 out]
            n152 = property on="stopTransport" class="Bool (strict)"("DisabledEnum"=w349) -> ()  [unwired: 2 in, 2 out]
            n153 = call <vilib>:"Add State(s) to Queue__jki_lib_state_machine.vi"("State(s) in (\"\")"=w364) -> ("States Out"=w363:string)  [unwired: 14 in]
          }
          frame "Data: Cleanup" {
            # "Cleanup any data and references, here.\n(this is called automatically, by the Macro: Exit)"
            n154 = Unbundle By Name(w375) -> ("Core.Current VI Reference"=w378:refnum<vi>)
            n155 = Close Reference(reference=w378, error in (no error)=w377) -> (error out=w376:errorcluster)
            n156 = call <vilib>:"Add State(s) to Queue__jki_lib_state_machine.vi"("State(s) in (\"\")"=w380) -> ("States Out"=w379:string)  [unwired: 14 in]
          }
          frame "---------- UI ----------" {
            # "Do not put any code in this frame.\n(It is a separator no-op. You can make a copy of this frame to create a new UI frame)"
            n157 = call <vilib>:"Add State(s) to Queue__jki_lib_state_machine.vi"("State(s) in (\"\")"=w385) -> ("States Out"=w384:string)  [unwired: 14 in]
          }
          frame "UI: Initialize" {
            # "Initialize the User Interface, here.\n(this is called automatically, by the Macro: Init)"
            n158 = call <userlib>:"Fit VI window to Largest Dec__ogtk.vi"("error in (no error)"=w388, "border spacing (2 px)"=0) -> ("error out"=w389:errorcluster)  [unwired: 4 in, 1 out]
            n159 = local write "Tab Control"(enum32{"Main", "Sweep Config", "Debug"}."Main" ("Tab Control")) -> ()
            n160 = property on="Ring" class="Ring (strict)"("Strings []"=string[] []) -> ()  [unwired: 2 in, 2 out]
            n161 = call <vilib>:"Add State(s) to Queue__jki_lib_state_machine.vi"("State(s) in (\"\")"=w394) -> ("States Out"=w393:string)  [unwired: 14 in]
          }
          frame "UI: Wait" {
            # "Do not put any code in this frame.\n(It is a separator no-op. You can make a copy of this frame to create a new UI frame)"
            n162 = Scan From String(format string="%d", input string=w395, default 1=u32 0 ("default value 1")) -> (output 1=w396:u32)  [unwired: 2 in, 3 out]
            n163 = Wait (ms)(milliseconds to wait=w396) -> ()  [unwired: 1 out]
            n164 = call <vilib>:"Add State(s) to Queue__jki_lib_state_machine.vi"("State(s) in (\"\")"=w403) -> ("States Out"=w402:string)  [unwired: 14 in]
          }
          frame "UI: Cursor Set" {
            # "Argument"
            # "Initialize the User Interface, here.\n(this is called automatically, by the Macro: Init)"
            n165 = disable-structure shown="Default" {
              disable-tunnel: w406 -> [w411 w414]
              disable-tunnel: [w411 w413] -> w405
              disable-tunnel: w404 -> [_ w412]
              frame condition #0 {
              }
              frame condition #1 (active) {
                n166 = case shown="\"Idle\", Default" w412 {
                  tunnel: w414 -> [w416 w418]
                  tunnel: [w415 w417] -> w413
                  frame "Idle", Default {
                    n167 = call <vilib>:"Unset Busy.vi"("error in (no error)"=w416) -> ("error out"=w415:errorcluster)  [unwired: 10 in]
                  }
                  frame "Busy" {
                    n168 = call <vilib>:"Set Busy.vi"("error in (no error)"=w418) -> ("error out"=w417:errorcluster)  [unwired: 9 in, 1 out]
                  }
                }
              }
            }
            n169 = call <vilib>:"Add State(s) to Queue__jki_lib_state_machine.vi"("State(s) in (\"\")"=w410) -> ("States Out"=w409:string)  [unwired: 14 in]
          }
          frame "UI: Front Panel State" {
            # "Argument"
            # "Set Front Panel Open or Closed\n(Usage: \"UI: Front Panel State >> Open|Close\")"
            n170 = Unbundle By Name(w422) -> ("Core.Current VI Reference"=w421:refnum<vi>)
            n171 = disable-structure shown="Default" {
              disable-tunnel: w424 -> [w430 w453]
              disable-tunnel: [w429 w453] -> w423
              disable-tunnel: w421 -> [w428 _]
              disable-tunnel: w420 -> [w427 _]
              frame condition #0 (active) {
                n172 = case shown="\"Open\", Default" w427 {
                  tunnel: w430 -> [w434 w447]
                  tunnel: [w436 w448] -> w429
                  tunnel: w428 -> [w435 w445]
                  frame "Open", Default {
                    n173 = property class="VI"(reference=w435, error in=w434) -> (reference out=w432:refnum<vi>, error out=w433:errorcluster, "FP.State"=w431:T10)
                    n174 = case shown="\"Closed\"" w431 {
                      tunnel: [w439 w442] -> w436
                      tunnel: w433 -> [w438 w442]
                      tunnel: w432 -> [w437 _]
                      frame "Closed" {
                        n175 = invoke class="VI" method="FP.Open"(reference=w437, error in=w438, "Activate"=TRUE, "State"=T10."Standard") -> (error out=w439:errorcluster)  [unwired: 1 in, 4 out]
                      }
                      frame Default {
                      }
                    }
                  }
                  frame "Close" {
                    n176 = property class="VI"(reference=w445, error in=w447) -> (reference out=w444:refnum<vi>, error out=w446:errorcluster, "FP.State"=w443:T10)
                    n177 = case shown="Default" w443 {
                      tunnel: [w449 w452] -> w448
                      tunnel: w446 -> [w449 w451]
                      tunnel: w444 -> [_ w450]
                      frame "Invalid", "Closed" {
                      }
                      frame Default {
                        n178 = invoke class="VI" method="FP.Close"(reference=w450, error in=w451) -> (error out=w452:errorcluster)  [unwired: 1 in, 2 out]
                      }
                    }
                  }
                }
              }
              frame condition #1 {
              }
            }
            n179 = call <vilib>:"Add State(s) to Queue__jki_lib_state_machine.vi"("State(s) in (\"\")"=w426) -> ("States Out"=w425:string)  [unwired: 14 in]
          }
          frame "UI: Transport Front Panel" {
            n180 = Unbundle By Name(w457) -> ("paths"=w459:path[], "Ring"=w454:i32)
            n181 = Index Array(array=w459, index=w454) -> (element=w455:path)
            n182 = Empty String/Path?(string/path=w455) -> (empty?=w456:bool)
            n183 = case shown="False" w456 {
              tunnel: [w472 w501] -> w461
              tunnel: w460 -> [w471 w501]
              tunnel: w458 -> [w470 _]
              tunnel: w455 -> [w465 _]
              frame False {
                n184 = Open VI Reference(vi path=w465, error in (no error)=w471) -> (vi reference=w468:refnum<vi>, error out=w469:errorcluster)  [unwired: 4 in]
                n185 = case shown="\"Close\"" w470 {
                  tunnel: w469 -> [w477 w493]
                  tunnel: [w479 w494] -> w466
                  tunnel: w468 -> [w478 w491]
                  tunnel: [w473 w488] -> w467
                  frame "Open", Default {
                    n186 = property class="VI"(reference=w478, error in=w477) -> (reference out=w475:refnum<vi>, error out=w476:errorcluster, "FP.State"=w474:T10)
                    n187 = case shown="\"Invalid\"" w474 {
                      tunnel: [w483 w487] -> w479
                      tunnel: w476 -> [w482 w487]
                      tunnel: w475 -> [w481 w486]
                      tunnel: [w480 w486] -> w473
                      frame Default {
                        n188 = invoke class="VI" method="FP.Open"(reference=w481, error in=w482, "Activate"=TRUE, "State"=T10."Standard") -> (reference out=w480:refnum<vi>, error out=w483:errorcluster)  [unwired: 1 in, 3 out]
                      }
                      frame "Invalid" {
                      }
                    }
                  }
                  frame "Close" {
                    n189 = property class="VI"(reference=w491, error in=w493) -> (reference out=w490:refnum<vi>, error out=w492:errorcluster, "FP.State"=w489:T10)
                    n190 = case shown="Default" w489 {
                      tunnel: [w496 w500] -> w494
                      tunnel: w492 -> [w496 w499]
                      tunnel: w490 -> [w495 w498]
                      tunnel: [w495 w497] -> w488
                      frame "Invalid", "Closed" {
                      }
                      frame Default {
                        n191 = invoke class="VI" method="FP.Close"(reference=w498, error in=w499) -> (reference out=w497:refnum<vi>, error out=w500:errorcluster)  [unwired: 1 in, 1 out]
                      }
                    }
                  }
                }
                n192 = Close Reference(reference=w467, error in (no error)=w466) -> (error out=w472:errorcluster)
              }
              frame True {
              }
            }
            n193 = call <vilib>:"Add State(s) to Queue__jki_lib_state_machine.vi"("State(s) in (\"\")"=w464) -> ("States Out"=w463:string)  [unwired: 14 in]
          }
          frame "---------- Macro ----------" {
            # "Do not put any code in this frame.\n(It is a separator no-op. You can make a copy of this frame to create a new Macro frame)"
            n194 = call <vilib>:"Add State(s) to Queue__jki_lib_state_machine.vi"("State(s) in (\"\")"=w506) -> ("States Out"=w505:string)  [unwired: 14 in]
          }
          frame "Macro: Initialize" {
            # "Initialization Macro\n(This is called once, when the VI starts)"
            n195 = call <vilib>:"Add State(s) to Queue__jki_lib_state_machine.vi"("State(s) in Front (\"\")"="Data: Initialize\nInitialize Core Data\nEvents: Register", "State(s) in (\"\")"="Process: Sync", "State(s) at Back (\"\")"="UI: Initialize\nUI: Front Panel State >> Close\nAction: Status >> Initializing...\nMacro: Debug\nData: Populate Ring\nAction: Status") -> ("States Out"=w510:string)  [unwired: 12 in]
            n196 = call <vilib>:"Add State(s) to Queue__jki_lib_state_machine.vi"("State(s) in Front (\"\")"=w510, "State(s) in (\"\")"=w515) -> ("States Out"=w514:string)  [unwired: 13 in]
          }
          frame "Macro: Post Error Handling" {
            # "Clear Last Error?"
            n197 = Unbundle By Name(w517) -> ("Core.Last Error.remaining states"=w519:string, "Core.Shutdown?"=w520:bool)
            n198 = Unbundle By Name(w517) -> ("Core.Last Error.error"=w523:errorcluster)
            n199 = case shown="False" FALSE {
              tunnel: w523 -> [w531 _]
              tunnel: [w531 _] -> w522
              frame False {
              }
              frame True {
              }
            }
            n200 = case shown="False" w520 {
              tunnel: w519 -> [w528 w530]
              tunnel: [w528 w529] -> w516
              frame False {
                # "These are the remaining states (at the moment the error occured). States can be altered according to business logic."
                # "NOT SHUTTING DOWN"
              }
              frame True {
                # "Developer can decide to alter the states but should be aware that during the shutdown process, there are certain states that must be run for the SMO to properly shut itself (and this process) down. As such, one can add states to perform additional clean-ups, but should append the remaining state to be executed."
                # "SHUTTING DOWN"
                n201 = call <vilib>:"Add State(s) to Queue__jki_lib_state_machine.vi"("State(s) in (\"\")"=w530) -> ("States Out"=w529:string)  [unwired: 14 in]
              }
            }
            n202 = Bundle By Name(cluster=w517, "Core.Last Error.error"=w522) -> (w518:T14)
            n203 = call <vilib>:"Add State(s) to Queue__jki_lib_state_machine.vi"("State(s) in Front (\"\")"=w516, "State(s) in (\"\")"=w527) -> ("States Out"=w526:string)  [unwired: 13 in]
          }
          frame "Macro: Run Sequence" {
            # "0,1,2,3,4,"
            # "5"
            # "Do not put any code in this frame.\n(It is a separator no-op. You can make a copy of this frame to create a new Macro frame)"
            n204 = Unbundle By Name(w538) -> ("sequence"=w534:string[], "Running Step"=w532:i32)
            n205 = Array Size(array=w534) -> (size(s)=w544:i32)
            n206 = Index Array(array=w534, index=w532) -> (element=w533:string)
            n207 = Greater Or Equal?(x=w544, y=w532) -> (x >= y?=w536:bool)
            n208 = Select(t=-1 ("Running Step"), s=w536, f=w532) -> (s? t:f=w543:i32)
            n209 = Bundle By Name(cluster=w538, "Running Step"=w543) -> (w539:T14)
            n210 = Select(t="Action: Status >> ...", s=w536, f="Idle //Check Event Structure\nMacro: Run Sequence" ("State(s) at Back (\"\")")) -> (s? t:f=w535:string)
            n211 = call <vilib>:"Add State(s) to Queue__jki_lib_state_machine.vi"("State(s) in Front (\"\")"=w533, "State(s) at Back (\"\")"=w535) -> ("States Out"=w537:string)  [unwired: 13 in]
            n212 = call <vilib>:"Add State(s) to Queue__jki_lib_state_machine.vi"("State(s) in Front (\"\")"=w537, "State(s) in (\"\")"=w548) -> ("States Out"=w547:string)  [unwired: 13 in]
          }
          frame "Macro: Debug" {
            # "exe?"
            # "If pane is an EXE, then close it when we exit"
            # "Macro: Debug\n(get debug behavior, determine UI and determine shutdown behavior)"
            n213 = Unbundle By Name(w552) -> ("Core.Close Panel on Exit?"=w555:bool, "SMO"=w560:refnum<class "Inst.Transport.lvclass">)
            n214 = property class="App"() -> ("App.Kind"=w558:T7)  [unwired: 2 in, 2 out]
            n215 = Equal?(x=w558, y=T7."Run Time System" ("Application:Kind")) -> (x = y?=w554:bool)
            n216 = call <userlib>:"Get Debug Mode.vi"("error in (no error)"=w550, "SMO"=w560) -> ("error out"=w551:errorcluster, "Behavior"=w559:T16)  [unwired: 7 in, 1 out]
            n217 = case shown="\"Debug\"" w559 {
              tunnel: [w564 w566] -> w556
              tunnel: w555 -> [w564 _]
              tunnel: w554 -> [_ w568]
              tunnel: [_ "UI: Front Panel State >> Open\nUI: Wait >> 1000"] -> w549
              frame "Normal", Default {
                # "respect core.close"
              }
              frame "Debug" {
                # "keep panel open\nunless exe"
                n218 = Or(x=w568, y=FALSE) -> (x .or. y?=w566:bool)
              }
            }
            n219 = Bundle By Name(cluster=w552, "Core.Close Panel on Exit?"=w556) -> (w553:T14)
            n220 = call <vilib>:"Add State(s) to Queue__jki_lib_state_machine.vi"("State(s) in Front (\"\")"=w549, "State(s) in (\"\")"=w563) -> ("States Out"=w562:string)  [unwired: 13 in]
          }
          frame "Macro: startTransport" {
            # "\"Macro: Start Transport\" \n()"
            n221 = call <vilib>:"Add State(s) to Queue__jki_lib_state_machine.vi"("State(s) in Front (\"\")"="Transport: prepareTransport\nTransport: startTransport" ("State(s) in Front (\"\")"), "State(s) in (\"\")"=w574) -> ("States Out"=w573:string)  [unwired: 13 in]
          }
          frame "Macro: Exit" {
            # "Exit Macro\n(This is called once, when the VI exits)"
            n222 = Unbundle By Name(w576) -> ("Core.Close Panel on Exit?"=w589:bool)
            n223 = Select(t="UI: Front Panel State >> Close", s=w589, f="" ("Empty String Constant")) -> (s? t:f=w587:string)
            n224 = Bundle By Name(cluster=w576, "Core.Shutdown?"=TRUE) -> (w577:T14)
            n225 = call <vilib>:"Add State(s) to Queue__jki_lib_state_machine.vi"("State(s) in Front (\"\")"="Data: Cleanup\nEvents: Unregister\n//Process: Self Terminate", "State(s) in (\"\")"="Process: Sync", "State(s) at Back (\"\")"="Exit") -> ("States Out"=w582:string)  [unwired: 12 in]
            n226 = call <vilib>:"Add State(s) to Queue__jki_lib_state_machine.vi"("State(s) in Front (\"\")"="Action: Status >> Shutting down...", "State(s) in (\"\")"=w587, "State(s) at Back (\"\")"=w582) -> ("States Out"=w586:string)  [unwired: 12 in]
            n227 = call <vilib>:"Add State(s) to Queue__jki_lib_state_machine.vi"("State(s) in Front (\"\")"=w586, "State(s) in (\"\")"=w591) -> ("States Out"=w590:string)  [unwired: 13 in]
          }
          frame "---------- Process ----------" {
            # "Template Separator\n(You can make a copy of, or modify, this frame)"
            n228 = call <vilib>:"Add State(s) to Queue__jki_lib_state_machine.vi"("State(s) in (\"\")"=w596) -> ("States Out"=w595:string)  [unwired: 14 in]
          }
          frame "Process: Sync" {
            n229 = Unbundle By Name(w604) -> ("SMO"=w600:refnum<class "Inst.Transport.lvclass">)
            n230 = call <vilib>:"WaitOnProcessSync.vi"("error in (no error)"=w599, "SMO"=w600) -> ("error out"=w598:errorcluster, "Don't run?"=w603:bool)  [unwired: 7 in, 1 out]
            n231 = Select(t="Data: Cleanup\nEvents: Unregister\nExit", s=w603, f="" ("Empty String Constant")) -> (s? t:f=w597:string)
            n232 = call <vilib>:"Add State(s) to Queue__jki_lib_state_machine.vi"("State(s) in Front (\"\")"=w597, "State(s) in (\"\")"=w607) -> ("States Out"=w606:string)  [unwired: 13 in]
          }
          frame "Process: Self Terminate" {
            # "Template Separator\n(You can make a copy of, or modify, this frame)"
            n233 = Unbundle By Name(w611) -> ("SMO"=w610:refnum<class "Inst.Transport.lvclass">)
            n234 = call <vilib>:"SelfTerminate.vi"("error in (no error)"=w608, "SMO in"=w610) -> ("error out"=w609:errorcluster)  [unwired: 8 in, 1 out]
            n235 = call <vilib>:"Add State(s) to Queue__jki_lib_state_machine.vi"("State(s) in (\"\")"=w614) -> ("States Out"=w613:string)  [unwired: 14 in]
          }
          frame "---------- Events ----------" {
            # "Template Separator\n(You can make a copy of, or modify, this frame)"
            n236 = call <vilib>:"Add State(s) to Queue__jki_lib_state_machine.vi"("State(s) in (\"\")"=w619) -> ("States Out"=w618:string)  [unwired: 14 in]
          }
          frame "Events: Register" {
            n237 = Unbundle By Name(w625) -> ("SMO"=w626:refnum<class "Inst.Transport.lvclass">)
            n238 = call <vilib>:"GetProtectedEvents.vi"("SMO"=w626) -> ("error out"=w624:errorcluster, "SMO Protected Events"=w629:T17, "SMO out"=w623:refnum<class "Inst.Transport.lvclass">)  [unwired: 8 in]
            n239 = call "Inst.Transport.GetPrivateEvents.vi"("Inst.Transport in"=w623) -> ("error out"=w620:errorcluster, "Transport Private Events"=w621:cluster{"MessageToProcess":refnum<user-event>})  [unwired: 8 in, 1 out]
            n240 = register-events(w629, w621) -> (reference out=w630:refnum<event-registration>, error out=w627:errorcluster)  [unwired: 2 in]
            n241 = Merge Errors(w627, w620, w624, w622) -> (w628:errorcluster)
            n242 = call <vilib>:"Add State(s) to Queue__jki_lib_state_machine.vi"("State(s) in (\"\")"=w632) -> ("States Out"=w631:string)  [unwired: 14 in]
          }
          frame "Events: Unregister" {
            n243 = Unregister For Events(event registration refnum=w635, error in=w634) -> (error out=w633:errorcluster)
            n244 = call <vilib>:"Clear Errors.vi"("error in (no error)"=w633) -> ()  [unwired: 5 in, 2 out]
            n245 = call <vilib>:"Add State(s) to Queue__jki_lib_state_machine.vi"("State(s) in (\"\")"=w638) -> ("States Out"=w637:string)  [unwired: 14 in]
          }
          frame "---------- Transport ----------" {
            n246 = Unbundle By Name(w641) -> ("SMO"=w639:refnum<class "Inst.Transport.lvclass">, "Transport"=w640:refnum<class "Transport.lvclass">)
            n247 = Bundle By Name(cluster=w641, "SMO"=w639, "Transport"=w640) -> (w642:T14)
            n248 = call <vilib>:"Add State(s) to Queue__jki_lib_state_machine.vi"("State(s) in (\"\")"=w646) -> ("States Out"=w645:string)  [unwired: 14 in]
          }
          frame "Transport: prepareTransport" {
            n249 = Unbundle By Name(w669) -> ("SMO"=w668:refnum<class "Inst.Transport.lvclass">, "Transport"=w653:refnum<class "Transport.lvclass">, "C.E."=w655:refnum<class "Control Experiment.lvclass">, "Comments"=w657:string, "Folder"=w656:string)
            n250 = call "Control Experiment FGV.vi"("Function"=enum16{"read", "write"}."read", "error in (no error)"=w660, "Control Experiment.lvclass"=refnum<class "Control Experiment.lvclass"> refnum) -> ("error out"=w664:errorcluster, "Control Experiment.lvclass out"=w666:refnum<class "Control Experiment.lvclass">)  [unwired: 5 in, 2 out]
            n251 = call "Write Experiment Folder.vi"("error in (no error)"=w664, "Experiment Folder"=w656, "Control Experiment in"=w666) -> ("error out"=w663:errorcluster, "Control Experiment out"=w665:refnum<class "Control Experiment.lvclass">)  [unwired: 7 in]
            n252 = call "Read All Dictionary Elements.vi"("Control Experiment in"=w655) -> ("Items"=w654:T18[])  [unwired: 8 in, 2 out]
            n253 = call "Write Experiment Description.vi"("error in (no error)"=w663, "Experiment Description"=w657, "Control Experiment in"=w665) -> ("error out"=w659:errorcluster, "Control Experiment out"=w662:refnum<class "Control Experiment.lvclass">)  [unwired: 7 in]
            n254 = call "Write Dictionary Elements (Loop).vi"("error in (no error)"=w659, "Data in"=w654, "Control Experiment in"=w662) -> ("error out"=w658:errorcluster, "Control Experiment out"=w661:refnum<class "Control Experiment.lvclass">)  [unwired: 7 in]
            n255 = call "Write Dependencies.vi"("error in (no error)"=w658, "Control Experiment"=w661, "Transport in"=w653) -> ("error out"=w649:errorcluster, "Transport out"=w651:refnum<class "Transport.lvclass">)  [unwired: 7 in]
            n256 = call "Send Stop Notifier.vi"("error in (no error)"=w649, "Stop [T]"=FALSE, "Transport in"=w651) -> ("error out"=w648:errorcluster, "Transport out"=w650:refnum<class "Transport.lvclass">)  [unwired: 7 in]
            n257 = Bundle By Name(cluster=w669, "SMO"=w668, "Transport"=w650) -> (w670:T14)
            n258 = call <vilib>:"Add State(s) to Queue__jki_lib_state_machine.vi"("State(s) in (\"\")"=w673) -> ("States Out"=w672:string)  [unwired: 14 in]
          }
          frame "Transport: startTransport" {
            n259 = Unbundle By Name(w680) -> ("Transport"=w679:refnum<class "Transport.lvclass">, "Ring"=w678:i32, "Status"=w674:T8)
            n260 = case shown="\"running\"" w674 {
              tunnel: w679 -> [_ w692]
              tunnel: [w686 "" ("State with Arguments")] -> w675
              tunnel: w676 -> [w684 w690]
              tunnel: [w684 w689] -> w677
              tunnel: w678 -> [_ w688]
              frame "running" {
                n261 = call <vilib>:"Build State String with Arguments__JKI_lib_State_Machine.vi"("Arguments (\"\")"="Experiment already running" ("Arguments (\"\")"), "State"="Action: Status") -> ("State with Arguments"=w686:string)  [unwired: 4 in]
              }
              frame "idle" {
                n262 = call "Transport.CallByReference.vi"("error in (no error)"=w690, "method"=w688, "Transport"=w692) -> ("error out"=w689:errorcluster)  [unwired: 8 in]
              }
            }
            n263 = call <vilib>:"Add State(s) to Queue__jki_lib_state_machine.vi"("State(s) in Front (\"\")"=w675, "State(s) in (\"\")"=w683) -> ("States Out"=w682:string)  [unwired: 13 in]
          }
          frame "Transport: stopTransport" {
            n264 = Unbundle By Name(w698) -> ("Transport"=w697:refnum<class "Transport.lvclass">)
            n265 = call "Send Stop Notifier.vi"("error in (no error)"=w694, "Stop [T]"=TRUE, "Transport in"=w697) -> ("error out"=w695:errorcluster, "Transport out"=w696:refnum<class "Transport.lvclass">)  [unwired: 7 in]
            n266 = Bundle By Name(cluster=w698, "Transport"=w696) -> (w699:T14)
            n267 = call <vilib>:"Add State(s) to Queue__jki_lib_state_machine.vi"("State(s) in (\"\")"=w702) -> ("States Out"=w701:string)  [unwired: 14 in]
          }
          frame "Transport: appendExptParam" {
            n268 = Unbundle By Name(w711) -> ("C.E."=w710:refnum<class "Control Experiment.lvclass">, "MessageToProcess.Message.Data"=w703:variant)
            n269 = call "Parse ExptParam.vi"("error in (no error)"=w705, "params in"=w703) -> ("error out"=w704:errorcluster, "value"=w706:variant, "key"=w707:string)  [unwired: 7 in]
            n270 = call "Append Dictionary Element.vi"("error in (no error)"=w704, "value"=w706, "key"=w707, "Control Experiment in"=w710) -> ("error out"=w708:errorcluster, "Control Experiment out"=w709:refnum<class "Control Experiment.lvclass">)  [unwired: 6 in]
            n271 = Bundle By Name(cluster=w711, "C.E."=w709) -> (w712:T14)
            n272 = call <vilib>:"Add State(s) to Queue__jki_lib_state_machine.vi"("State(s) in (\"\")"=w715) -> ("States Out"=w714:string)  [unwired: 14 in]
          }
          frame "Transport: setExptParam" {
            n273 = Unbundle By Name(w724) -> ("C.E."=w723:refnum<class "Control Experiment.lvclass">, "MessageToProcess.Message.Data"=w720:variant)
            n274 = call "Parse ExptParam.vi"("error in (no error)"=w719, "params in"=w720) -> ("error out"=w718:errorcluster, "value"=w716:variant, "key"=w717:string)  [unwired: 7 in]
            n275 = call "Write Dictionary Element.vi"("error in (no error)"=w718, "value"=w716, "key"=w717, "Control Experiment in"=w723) -> ("error out"=w721:errorcluster, "Control Experiment out"=w722:refnum<class "Control Experiment.lvclass">)  [unwired: 6 in]
            n276 = Bundle By Name(cluster=w724, "C.E."=w722) -> (w725:T14)
            n277 = call <vilib>:"Add State(s) to Queue__jki_lib_state_machine.vi"("State(s) in (\"\")"=w728) -> ("States Out"=w727:string)  [unwired: 14 in]
          }
          frame "Transport: clearExptParam" {
            n278 = Bundle By Name(cluster=w730, "C.E."=refnum<class "Control Experiment.lvclass"> refnum) -> (w731:T14)
            n279 = call <vilib>:"Add State(s) to Queue__jki_lib_state_machine.vi"("State(s) in (\"\")"=w735) -> ("States Out"=w734:string)  [unwired: 14 in]
          }
          frame "Transport: setSweepConfig" {
            n280 = Unbundle By Name(w741) -> ("Transport"=w739:refnum<class "Transport.lvclass">, "Sweep"=w737:T1)
            n281 = call "Write Configure Sweep.vi"("error in (no error)"=w736, "Lockin_Sweep"=w737, "Transport in"=w739) -> ("error out"=w738:errorcluster, "Transport out"=w740:refnum<class "Transport.lvclass">)  [unwired: 7 in]
            n282 = Bundle By Name(cluster=w741, "Transport"=w740) -> (w742:T14)
            n283 = call <vilib>:"Add State(s) to Queue__jki_lib_state_machine.vi"("State(s) in (\"\")"=w745) -> ("States Out"=w744:string)  [unwired: 14 in]
          }
          frame "Transport: setRefreshTime" {
            n284 = Unbundle By Name(w755) -> ("Transport"=w750:refnum<class "Transport.lvclass">, "MessageToProcess.Message.Data"=w747:variant)
            n285 = call "JSON to LVtype.vim"("type"=T11 {"RefreshTime"=0} ("setRefreshTime"), "error in (no error)"=w754, "JSON Data in"=w747) -> ("error out"=w753:errorcluster, "Data out"=w746:T11)  [unwired: 7 in]
            n286 = Unbundle By Name(w746) -> ("RefreshTime"=w749:u32)
            n287 = call "Send RefreshTime Notifier.vi"("error in (no error)"=w753, "RefreshTime (ms)"=w749, "Transport in"=w750) -> ("error out"=w752:errorcluster, "Transport out"=w751:refnum<class "Transport.lvclass">)  [unwired: 7 in]
            n288 = Bundle By Name(cluster=w755, "Transport"=w751) -> (w756:T14)
            n289 = call <vilib>:"Add State(s) to Queue__jki_lib_state_machine.vi"("State(s) in (\"\")"=w759) -> ("States Out"=w758:string)  [unwired: 14 in]
          }
          frame "Transport: Log" {
            # "THIS process.vi is responsible for logging data. Logging can be triggered in the timeout (as shown in this template proces.vi's tieout case) OR it could be triggered by data changes, or any other way you can device.\n\nThe code above will log ALL data. But you have the ability to log a subset, log some items on a different schedule, etc."
            n290 = Unbundle By Name(w768) -> ("SMO"=w764:refnum<class "Inst.Transport.lvclass">)
            n291 = call-dynamic "Get SMO Database Paths.vi"("error in (no error)"=w761, "Inst.Transport in"=w764) -> ("error out"=w762:errorcluster, "Paths"=w765:string, "Inst.Transport out"=w760:refnum<class "Inst.Transport.lvclass">)  [unwired: 7 in]
            n292 = Unbundle By Name(w760) -> ("Data"=w763:T19)
            n293 = call <userlib>:"Instrument.logToDatabase.vi"("error in (no error)"=w762, "Data"=w763, "Paths"=w765, "Instrument"=w760) -> ("error out"=w766:errorcluster, "Instrument out"=w767:refnum<class "Inst.Transport.lvclass">)  [unwired: 6 in]
            n294 = Bundle By Name(cluster=w768, "SMO"=w767) -> (w769:T14)
            n295 = call <vilib>:"Add State(s) to Queue__jki_lib_state_machine.vi"("State(s) in (\"\")"=w772) -> ("States Out"=w771:string)  [unwired: 14 in]
          }
          frame "---------- Action ----------" {
            n296 = call <vilib>:"Add State(s) to Queue__jki_lib_state_machine.vi"("State(s) in (\"\")"=w777) -> ("States Out"=w776:string)  [unwired: 14 in]
          }
          frame "Action: UI Status" {
            n297 = Unbundle By Name(w782) -> ("SMO"=w785:refnum<class "Inst.Transport.lvclass">)
            n298 = Unbundle By Name(w785) -> ("UI State"=w784:refnum<user-event>)
            n299 = Scan From String(input string=w781, default 1=UI_State--enum."Closed" ("event data")) -> (output 1=w778:T2)  [unwired: 3 in, 3 out]
            n300 = Generate User Event(user event=w784, event data cluster=w778, error in=w779) -> (error out=w780:errorcluster)  [unwired: 1 in, 1 out]
            n301 = call <vilib>:"Add State(s) to Queue__jki_lib_state_machine.vi"("State(s) in (\"\")"=w788) -> ("States Out"=w787:string)  [unwired: 14 in]
          }
          frame "Action: Status" {
            # "Sequence: Status\n(Use this frame to pass the status to the UI, this VI's UI, etc)"
            n302 = call <vilib>:"Add State(s) to Queue__jki_lib_state_machine.vi"("State(s) in (\"\")"=w794) -> ("States Out"=w793:string)  [unwired: 14 in]
            "Secret Status" <- w789
            "Status" <- w789
          }
          frame "Action: Wait" {
            # "Sequence: Wait\n(Non-Blocking Wait)"
            # "F = repeat this state. wait\nT = go to next state. don't wait"
            n303 = Unbundle By Name(w803) -> ("Running Step"=w796:i32)
            n304 = call <userlib>:"Wait Logic.vi"("error in (no error)"=w799, "Time"=w797) -> ("error out"=w798:errorcluster, "Status String"=w795:string, "Trigger"=w800:bool)  [unwired: 6 in, 1 out]
            n305 = Increment(x=w796) -> (x+1=w810:i32)
            n306 = Select(t=w810, s=w800, f=w796) -> (s? t:f=w801:i32)
            n307 = Select(t=u32 0, s=w800, f=u32 100 ("milliseconds to wait")) -> (s? t:f=w807:u32)
            n308 = call <userlib>:"Wait (ms)__ogtk.vi"("error in (no error)"=w798, "milliseconds to wait"=w807) -> ("error out"=w805:errorcluster)  [unwired: 8 in, 1 out]
            n309 = Bundle By Name(cluster=w803, "Running Step"=w801) -> (w802:T14)
            n310 = call <vilib>:"Build State String with Arguments__JKI_lib_State_Machine.vi"("Arguments (\"\")"=w795, "State"="Action: Status") -> ("State with Arguments"=w804:string)  [unwired: 4 in]
            n311 = call <vilib>:"Add State(s) to Queue__jki_lib_state_machine.vi"("State(s) in Front (\"\")"=w804, "State(s) in (\"\")"=w813) -> ("States Out"=w812:string)  [unwired: 13 in]
          }
        }
      }
    }
    frame Error {
    }
  }
  n312 = call-parent "Process.vi"("error in"=w3, "Instrument"=w6) -> ("error out"=w5:errorcluster, "Instrument out"=→"Inst.Transport out":refnum<class "Inst.Transport.lvclass">)  [unwired: 8 in]
  n313 = Merge Errors(w5, w4) -> (→"error out":errorcluster)
